vi "RFSA 5668 Scanning Speed Benchmark.vi"() -> ()   [LabVIEW 2017]
doc: "Demonstrates the basics of spectrum acquisition using the RF vector signal analyzer. The example shows how to configure the <B>Clock Source</B>, <B>Reference Level</B>, <B>Start Frequency</B>, <B>Stop Frequency</B>, <B>Resolution Bandwidth</B>, and the spectrum acquisition type parameters. This example plots the acquired Power Spectrum data on the graph."
uses:
  <instrlib>/niRFSA/niRFSA.llb/niRFSA Ref Clock Sources.ctl
  <vilib>/Utility/error.llb/DialogType.ctl
  <instrlib>/niRFSA/niRFSA.llb/niRFSA Read Power Spectrum (DBL).vi
panel:
  in  "Frequency Settling":dbl=1.0 format="%#_6f"
  in  "Clock Source":T1="OnboardClock"
  in  "Resource Name":refnum<k15>="RFSA"
  out "Power Spectrum":cluster{"f0":dbl, "df":dbl, "data":dbl[]}(graph)
  in  "Stop Frequency (Hz)":dbl=1010000000.0 format="%#.3p"
  in  "Start Frequency (Hz)":dbl=990000000.0 format="%#.3p"
  in  "Reference Level (dBm)":dbl format="%.2f"
  in  "Resolution Bandwidth (Hz)":dbl=10000.0 format="%#.3p"
  # "Overview: Demonstrates the basics of spectrum acquisition using the RF vector signal analyzer. \nRequirements: NI-RFSA\nInstructions:\n1. Change the Resource Name to your device.\n2. Run the VI."
  # "If you configure a span (Stop Frequency and Start Frequency) larger than the instantaneous bandwidth of the device, NI-RFSA automatically performs multiple acquisitions and combines them into a single spectrum."
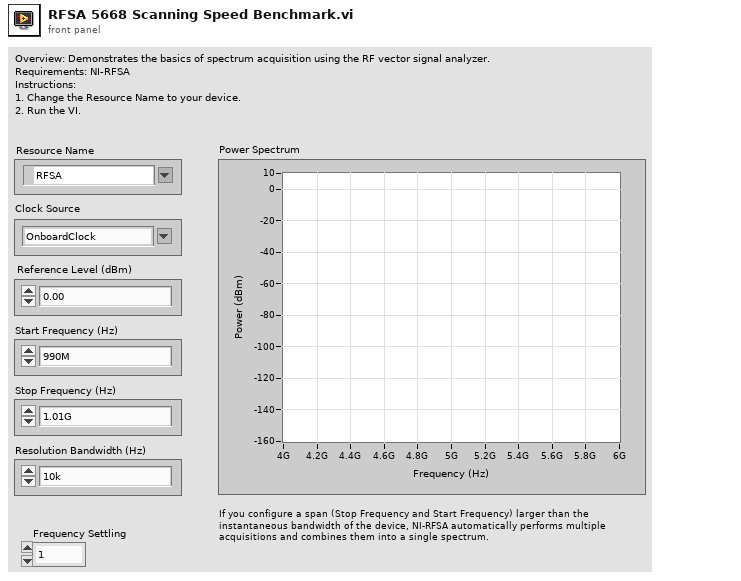
[diagram p1: front panel]
types:
  T1 = typedef "niRFSA Ref Clock Sources.ctl" = string
  T2 = typedef "DialogType.ctl" = u16
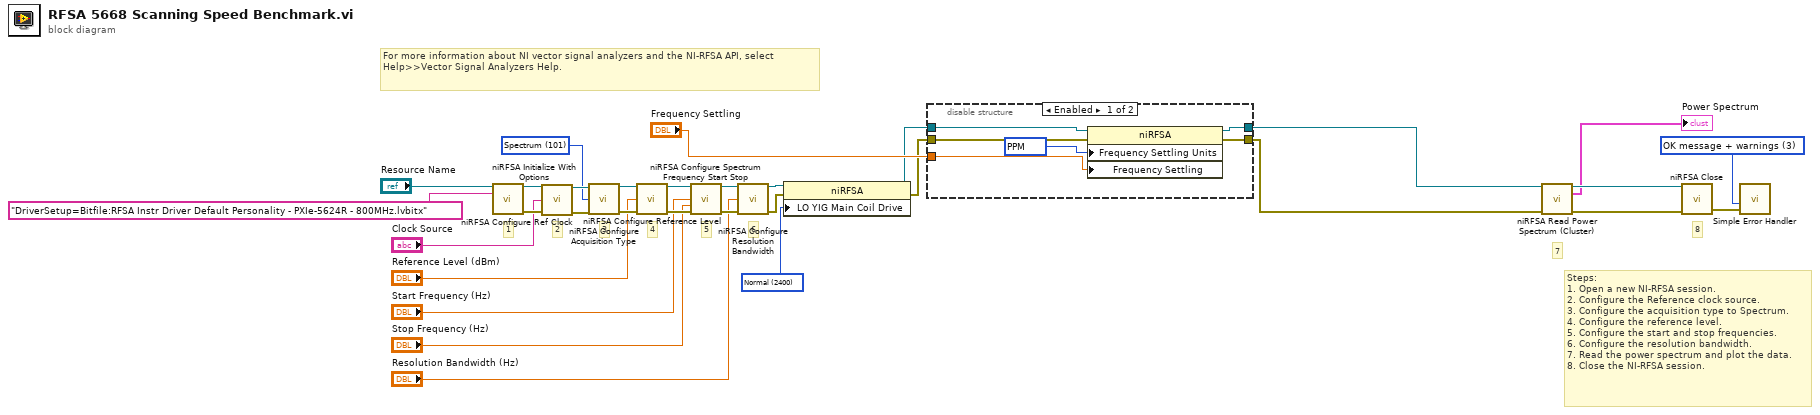
[diagram p0: block diagram]
diagram:
  w1 = 2400 items=["Normal"=2400, "Fast"=2401] ("Signal Path:Advanced:LO YIG Main Coil Drive")
  w12 = T2 3 items=["no dialog", "OK message", "continue or stop message", "OK message + warnings", "continue/stop + warnings"] ("type of dialog (OK msg:1)")
  w17 = 101 items=["IQ"=100, "Spectrum"=101] ("Acquisition:Acquisition Type")
  # "For more information about NI vector signal analyzers and the NI-RFSA API, select                                      Help>>Vector Signal Analyzers Help."
  # "2"
  # "Steps:\n1. Open a new NI-RFSA session.\n2. Configure the Reference clock source.\n3. Configure the acquisition type to Spectrum.\n4. Configure the reference level.\n5. Configure the start and stop frequencies.\n6. Configure the resolution bandwidth.\n7. Read the power spectrum and plot the data.\n8. Close the NI-RFSA session."
  # "8"
  # "7"
  # "6"
  # "5"
  # "4"
  # "3"
  # "1"
  n1 = call <instrlib>:"niRFSA Initialize With Options.vi"("resource name"="Resource Name", "option string"="DriverSetup=Bitfile:RFSA Instr Driver Default Personality - PXIe-5624R - 800MHz.lvbitx") -> ("instrument handle out"=w21:refnum<k15>, "error out"=w22:errorcluster)  [unwired: 12 in]
  n2 = call <instrlib>:"niRFSA Configure Ref Clock.vi"("instrument handle"=w21, "clock source"="Clock Source", "error in"=w22) -> ("instrument handle out"=w20:refnum<k15>, "error out"=w19:errorcluster)  [unwired: 11 in]
  n3 = call <instrlib>:"niRFSA Configure Acquisition Type.vi"("instrument handle"=w20, "acquisition type"=w17, "error in"=w19) -> ("instrument handle out"=w25:refnum<k15>, "error out"=w26:errorcluster)  [unwired: 11 in]
  n4 = call <instrlib>:"niRFSA Configure Reference Level.vi"("instrument handle"=w25, "reference level (dBm)"="Reference Level (dBm)", "error in"=w26) -> ("instrument handle out"=w31:refnum<k15>, "error out"=w30:errorcluster)  [unwired: 11 in]
  n5 = call <instrlib>:"niRFSA Configure Spectrum Frequency Start Stop.vi"("instrument handle"=w31, "start frequency"="Start Frequency (Hz)", "stop frequency"="Stop Frequency (Hz)", "error in"=w30) -> ("instrument handle out"=w24:refnum<k15>, "error out"=w23:errorcluster)  [unwired: 10 in]
  n6 = call <instrlib>:"niRFSA Configure Resolution Bandwidth.vi"("instrument handle"=w24, "resolution bandwidth (Hz)"="Resolution Bandwidth (Hz)", "error in"=w23) -> ("instrument handle out"=w5:refnum<k15>, "error out"=w2:errorcluster)  [unwired: 11 in]
  n7 = property class="niRFSA"(reference=w5, error in=w2, "LO YIG Main Coil Drive"=w1) -> (reference out=w4:refnum<k15>, error out=w3:errorcluster)
  n8 = disable-structure shown="Enabled" {
    disable-tunnel: w4 -> [w32 w39]
    disable-tunnel: w3 -> [w37 w38]
    disable-tunnel: [w36 w38] -> w7
    disable-tunnel: [w35 w39] -> w8
    disable-tunnel: "Frequency Settling" -> [w34 _]
    frame Enabled {
      w33 = 2000 items=["PPM"=2000, "Seconds After Lock"=2001, "Seconds After I/O"=2002] ("Signal Path:Advanced:Frequency Settling Units")
      n9 = property class="niRFSA"(reference=w32, error in=w37, "Frequency Settling Units"=w33, "Frequency Settling"=w34) -> (reference out=w35:refnum<k15>, error out=w36:errorcluster)
    }
    frame Disabled {
    }
  }
  n10 = call-poly <instrlib>:"niRFSA Read Power Spectrum (Cluster).vi"("instrument handle"=w8, "error in"=w7) -> ("instrument handle out"=w29:refnum<k15>, "power spectrum"=→"Power Spectrum":cluster{"f0":dbl, "df":dbl, "data":dbl[]}, "error out"=w27:errorcluster)  [unwired: 11 in]
  n11 = call <instrlib>:"niRFSA Close.vi"("instrument handle"=w29, "error in"=w27) -> ("error out"=w18:errorcluster)  [unwired: 13 in]
  n12 = call <vilib>:"Simple Error Handler.vi"("type of dialog (OK msg:1)"=w12, "error in (no error)"=w18) -> ()  [unwired: 3 in, 5 out]
